vi "Write ADU Packet.vi"(8 "error in":errorcluster, 9 "ELAN data unit":refnum<class "ELAN PDU.lvclass">, 10 "isMaster (f)":bool, 11 "ELAN data unit (ADU) in":refnum<class "ELAN Data Unit.lvclass">) -> (0 "error out":errorcluster, 3 "ELAN data unit (ADU) out":refnum<class "ELAN Data Unit.lvclass">)   [LabVIEW 2021, in "ELAN Data Unit.lvclass"]
uses:
  ELAN Data Unit.lvclass
  Data Unit/ELAN PC Data Unit/ELAN PDU.lvclass
  ELAN Data Unit.lvclass/ELAN Data Unit.ctl
  Data Unit/ELAN PC Data Unit/ELAN PDU.lvclass/ELAN PDU.ctl
  <vilib>/Utility/error.llb/Error Cluster From Error Code.vi
  <vilib>/ErrorRing/Error Ring.xnode
  Modbus_v121c/Network Interface/Serial Interface/Serial Shared Components/Serial Shared Components.lvlib
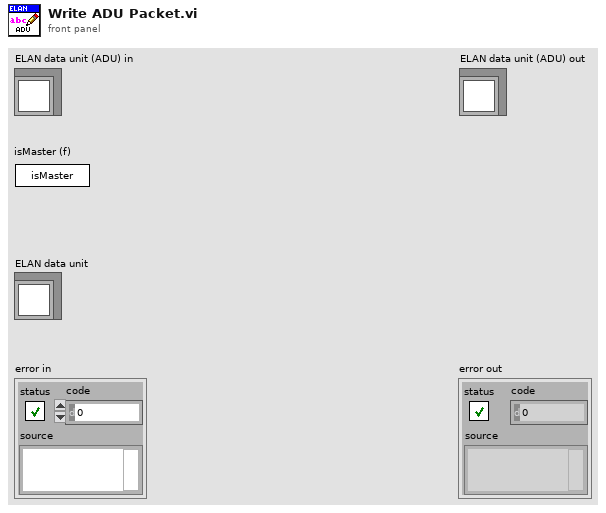
[diagram p1: front panel]
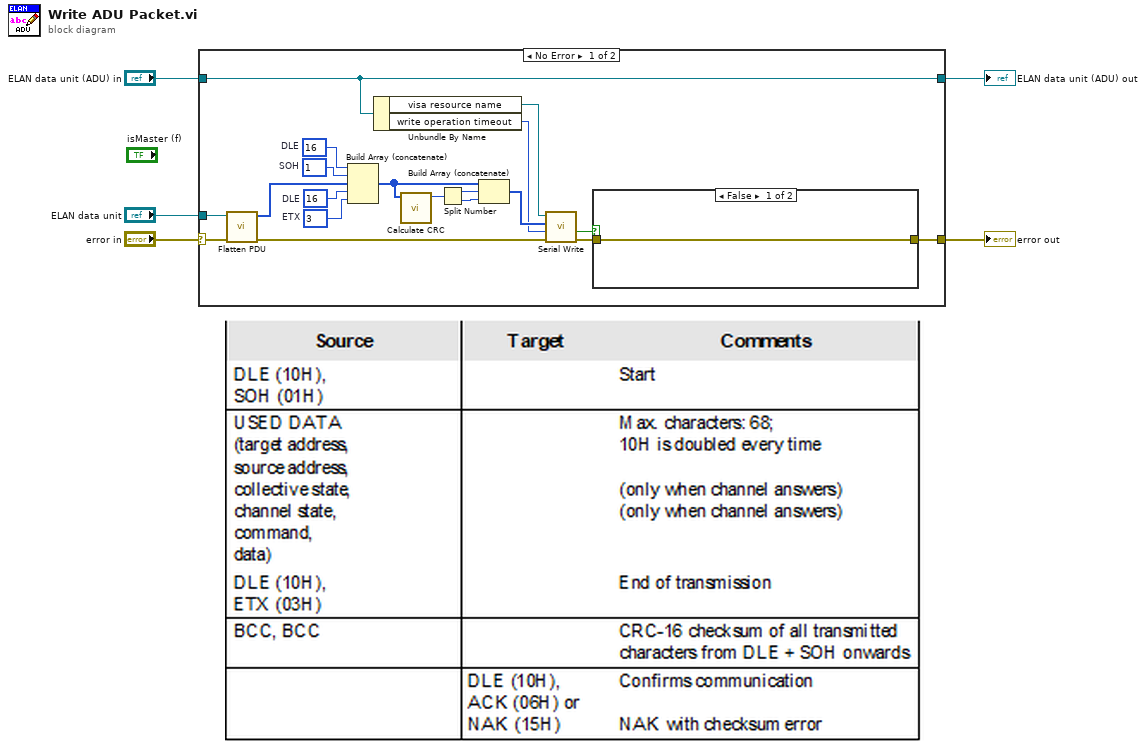
[diagram p0: block diagram]
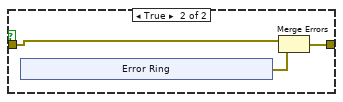
[diagram p2: hidden frame]
diagram:
  n1 = case shown="No Error" "error in" {
    selector: "error in" -> [w23 w34]
    tunnel: [w24 w34] -> w3
    tunnel: "ELAN data unit" -> [w22 _]
    tunnel: "ELAN data unit (ADU) in" -> [w8 w33]
    tunnel: [w8 w33] -> w4
    frame No Error {
      w10 = u8 16  # DLE
      w9 = u8 3  # ETX
      w12 = u8 16  # DLE
      w11 = u8 1  # SOH
      n2 = call "Flatten PDU.vi"("error in"=w23, "ELAN data unit in"=w22) -> ("error out"=w21:errorcluster, "Full ELAN data unit"=w18:u8[])  [unwired: 8 in]
      n3 = Build Array (concatenate)(w12, w11, w18, w10, w9) -> (w17:u8[])
      n4 = Unbundle By Name(w8) -> ("visa resource name"=w7:refnum<visa-resource-name>, "write operation timeout"=w6:u32)
      n5 = call "Calculate CRC.vi"("data"=w17) -> ("CRC-16"=w16:u16)  [unwired: 10 in]
      n6 = Split Number(x=w16) -> (hi(x)=w15:u8, lo(x)=w14:u8)
      n7 = Build Array (concatenate)(w17, w15, w14) -> (w13:u8[])
      n8 = call "Serial Write.vi"("error in"=w21, "timeout (ms)"=w6, "data"=w13, "Visa Resource"=w7) -> ("error out"=w19:errorcluster, "timed out?"=w20:bool)  [unwired: 6 in]
      n9 = case shown="False" w20 {
        tunnel: w19 -> [w25 w27]
        tunnel: [w25 w28] -> w24
        frame False {
        }
        frame True {
          n10 = xnode "Error Ring"() -> ("error out"=w26:errorcluster)
          n11 = Merge Errors(w27, w26) -> (w28:errorcluster)
        }
      }
    }
    frame Error {
    }
  }
  "error out" <- w3
  "ELAN data unit (ADU) out" <- w4
